vi "Manual.vi"(8 "error in (no error)":errorcluster, 10 "shutdown":refnum<user-event>, 11 "Modules":T2) -> (0 "Error 2":errorcluster)   [LabVIEW 2025]
uses:
  <vilib>/Handler Framework/CmdQueue/Enqueue Single.vi
  <vilib>/Handler Framework/Handler Framework.lvlib
  Libraries/USB IO/USB IO.lvlib
  Libraries/Wheatstone Bridge/Wheatstone Bridge.lvlib
  Libraries/Motor/Motor.lvlib
  Controls/Waveform Chart.ctl
panel:
  in  "Unit Power":bool
  in  "Brake Disable":bool
  in  "Position":dbl min=0.0 max=180.0
  out "Waveform Chart":T1
  out "Angle":dbl format="%5.3f°"
  out "Torque":dbl format="%5.3f lb-in"
  in  "Clear Motor Error":bool
  out "error out":errorcluster
  out "Module Names":string[](array[string])
  out "Error":errorcluster
  # "Manual"
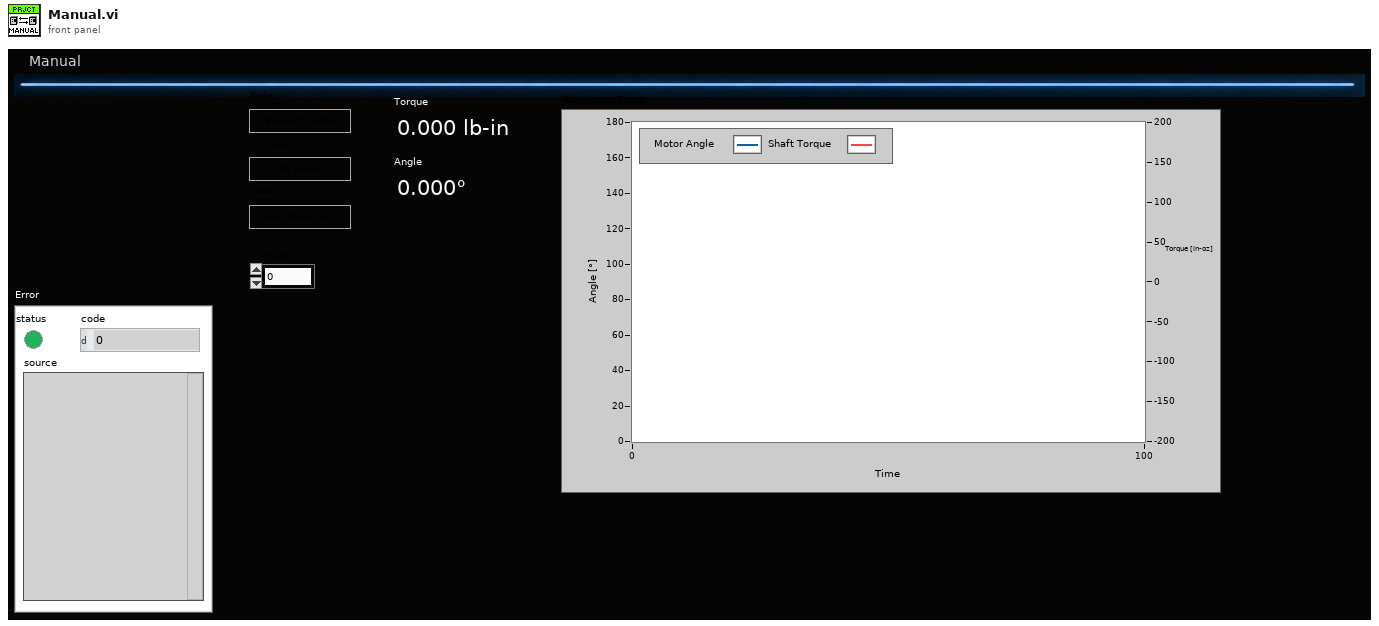
[diagram p1: front panel]
types:
  T1 = typedef "Waveform Chart.ctl" = dbl
  T2 = cluster{"Module IDs":i32[], "Module Names":string[]}
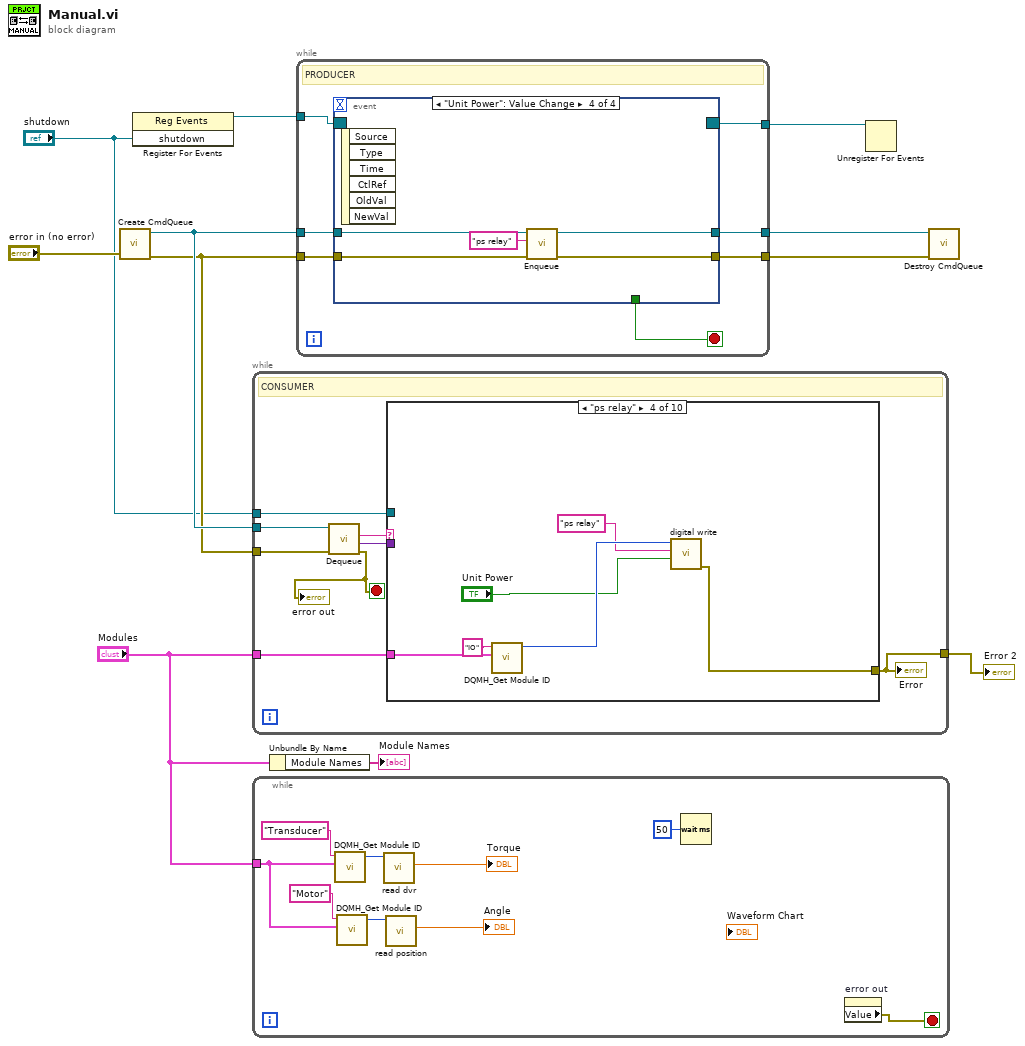
[diagram p0: block diagram]
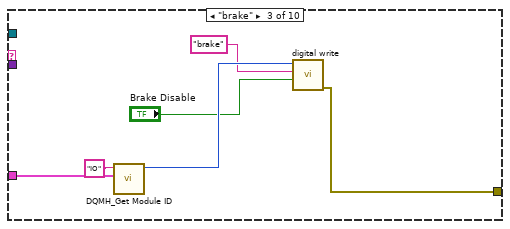
[diagram p4: hidden frame]
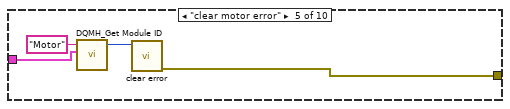
[diagram p5: hidden frame]
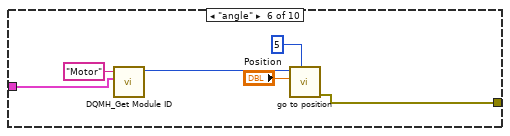
[diagram p6: hidden frame]
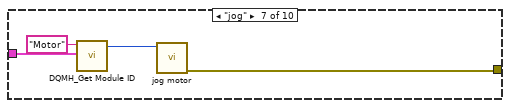
[diagram p7: hidden frame]
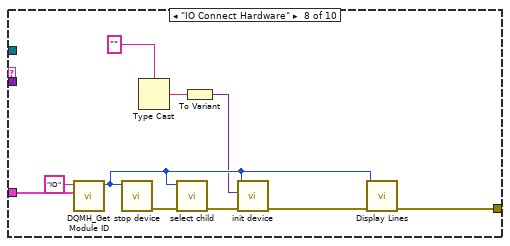
[diagram p8: hidden frame]
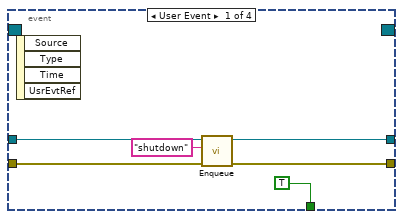
[diagram p11: hidden frame]
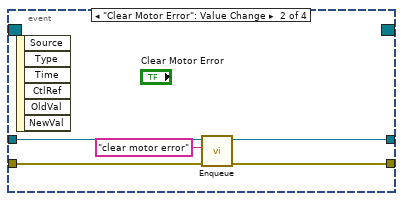
[diagram p12: hidden frame]
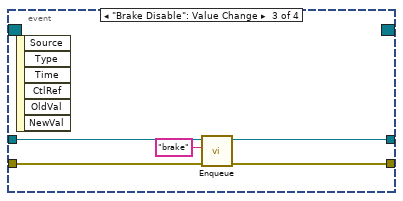
[diagram p13: hidden frame]
diagram:
  n1 = call <vilib>:"Create CmdQueue.vi"("error in (no error)"="error in (no error)") -> ("error out"=w8:errorcluster, "CmdQueue out"=w9:refnum<queue>)  [unwired: 9 in]
  n2 = register-events("shutdown") -> (reference out=w7:refnum<event-registration>)  [unwired: 2 in, 1 out]
  n3 = while {
    tunnel: w9 -> [w19]
    tunnel: w8 -> [w15]
    tunnel: "shutdown" -> [w14]
    tunnel: "Modules" -> [w13]
    tunnel: [w12] -> w2
    stop <- w16 stop-if-true
    # "CONSUMER"
    n4 = call <vilib>:"Dequeue.vi"("error in (no error)"=w15, "CmdQueue in"=w19) -> ("error out"=w16:errorcluster, "value"=w17:variant, "cmd"=w18:string)  [unwired: 5 in, 2 out]
    "error out" <- w16
    n5 = case shown="\"ps relay\"" w18 {
      tunnel: w17 -> [_ _ _ _ _ _ _ _ _ _]
      tunnel: w14 -> [_ _ _ _ _ _ _ _ _ _]
      tunnel: w13 -> [_ _ w24 w30 w34 w40 w45 w55 _ _]
      tunnel: [_ _ w22 w28 w32 w38 w42 w46 _ _] -> w12
      frame "False", Default {
      }
      frame "init" {
      }
      frame "brake" {
        n6 = call "DQMH_Get Module ID.vi"("Modules"=w24, "Module Name"="IO") -> ("Module ID out"=w23:i32)  [unwired: 9 in]
        n7 = call "digital write.vi"("On/Off"="Brake Disable", "Line"="brake", "Module ID"=w23) -> ("error out"=w22:errorcluster)  [unwired: 7 in, 1 out]
      }
      frame "ps relay" {
        n8 = call "DQMH_Get Module ID.vi"("Modules"=w30, "Module Name"="IO") -> ("Module ID out"=w29:i32)  [unwired: 9 in]
        n9 = call "digital write.vi"("On/Off"="Unit Power", "Line"="ps relay", "Module ID"=w29) -> ("error out"=w28:errorcluster)  [unwired: 7 in, 1 out]
      }
      frame "clear motor error" {
        n10 = call "DQMH_Get Module ID.vi"("Modules"=w34, "Module Name"="Motor") -> ("Module ID out"=w33:i32)  [unwired: 9 in]
        n11 = call "clear error.vi"("Module ID"=w33) -> ("error out"=w32:errorcluster)  [unwired: 9 in, 1 out]
      }
      frame "angle" {
        n12 = call "DQMH_Get Module ID.vi"("Modules"=w40, "Module Name"="Motor") -> ("Module ID out"=w39:i32)  [unwired: 9 in]
        n13 = call "go to position.vi"("Pause Time [ms]"=5, "Position"="Position", "Module ID"=w39) -> ("error out"=w38:errorcluster)  [unwired: 6 in, 2 out]
      }
      frame "jog" {
        n14 = call "DQMH_Get Module ID.vi"("Modules"=w45, "Module Name"="Motor") -> ("Module ID out"=w43:i32)  [unwired: 9 in]
        n15 = call "jog motor.vi"("Module ID"=w43) -> ("error out"=w42:errorcluster)  [unwired: 8 in, 2 out]
      }
      frame "IO Connect Hardware" {
        n16 = call "DQMH_Get Module ID.vi"("Modules"=w55, "Module Name"="IO") -> ("Module ID out"=w53:i32)  [unwired: 9 in]
        n17 = call "stop device.vi"("Module ID"=w53) -> ("error out"=w49:errorcluster)  [unwired: 9 in, 1 out]
        n18 = Type Cast(type="") -> (*(type *) &x=w51:string)  [unwired: 1 in]
        n19 = call "select child.vi"("error in"=w49, "Module ID"=w53) -> ("error out"=w47:errorcluster)  [unwired: 8 in, 1 out]
        n20 = To Variant(anything=w51) -> (Variant=w50:variant)
        n21 = call "init device.vi"("error in"=w47, "Variant"=w50, "Module ID"=w53) -> ("error out"=w48:errorcluster)  [unwired: 7 in, 1 out]
        n22 = call "Display Lines.vi"("error in"=w48, "Module ID"=w53) -> ("error out"=w46:errorcluster)  [unwired: 6 in, 3 out]
      }
      frame "Read Voltage" {
      }
      frame "shutdown" {
      }
    }
    "Error" <- w12
  }
  "Error 2" <- w2
  n23 = while {
    tunnel: "Modules" -> [w58]
    stop <- w62 stop-if-true
    n24 = call "DQMH_Get Module ID.vi"("Modules"=w58, "Module Name"="Transducer") -> ("Module ID out"=w63:i32)  [unwired: 9 in]
    n25 = call "DQMH_Get Module ID.vi"("Modules"=w58, "Module Name"="Motor") -> ("Module ID out"=w57:i32)  [unwired: 9 in]
    n26 = call "read dvr.vi"("Module ID"=w63) -> ("Numeric"=→"Torque":dbl)  [unwired: 8 in, 2 out]
    n27 = call "read position.vi"("Module ID"=w57) -> ("Position"=→"Angle":dbl)  [unwired: 8 in, 2 out]
    n28 = Wait (ms)(milliseconds to wait=u32 50) -> ()  [unwired: 1 out]
    n29 = property on="error out" class="Clust (strict)"() -> ("Value"=w62:errorcluster)  [unwired: 2 in, 2 out]
  }
  n30 = Unbundle By Name("Modules") -> ("Module Names"=→"Module Names":string[])
  n31 = while {
    tunnel: w9 -> [w71]
    tunnel: [w70] -> w11
    tunnel: w8 -> [w69]
    tunnel: [w68] -> w10
    tunnel: w7 -> [w66]
    tunnel: [w65] -> w6
    stop <- w67 stop-if-true
    # "PRODUCER"
    n32 = event shown="[3] \"Unit Power\": Value Change" {
      selector: w66 -> [_ _ _ _]
      dyn-events: [_ _ _ _] -> w65
      timeout: _ -> [_ _ _ _]
      tunnel: w71 -> [w77 w82 w87 w92]
      tunnel: [w76 w81 w86 w91] -> w70
      tunnel: w69 -> [w75 w80 w85 w90]
      tunnel: [w74 w79 w84 w89] -> w68
      tunnel: [TRUE ("Discard?") _ _ _] -> w67
      event User Event {
        n33 = event-data() -> ()  [unwired: 1 in, 4 out]
        n34 = call-poly <vilib>:"Enqueue.vi"("error in (no error)"=w75, "Command"="shutdown", "CmdQueue in"=w77) -> ("error out"=w74:errorcluster, "CmdQueue out"=w76:refnum<queue>)  [unwired: 7 in]
      }
      event "Clear Motor Error": Value Change {
        n35 = event-data() -> ()  [unwired: 1 in, 6 out]
        n36 = call-poly <vilib>:"Enqueue.vi"("error in (no error)"=w80, "Command"="clear motor error", "CmdQueue in"=w82) -> ("error out"=w79:errorcluster, "CmdQueue out"=w81:refnum<queue>)  [unwired: 7 in]
      }
      event "Brake Disable": Value Change {
        n37 = event-data() -> ()  [unwired: 1 in, 6 out]
        n38 = call-poly <vilib>:"Enqueue.vi"("error in (no error)"=w85, "Command"="brake", "CmdQueue in"=w87) -> ("error out"=w84:errorcluster, "CmdQueue out"=w86:refnum<queue>)  [unwired: 7 in]
      }
      event "Unit Power": Value Change {
        n39 = event-data() -> ()  [unwired: 1 in, 6 out]
        n40 = call-poly <vilib>:"Enqueue.vi"("error in (no error)"=w90, "Command"="ps relay", "CmdQueue in"=w92) -> ("error out"=w89:errorcluster, "CmdQueue out"=w91:refnum<queue>)  [unwired: 7 in]
      }
    }
  }
  n41 = Unregister For Events(event registration refnum=w6) -> ()  [unwired: 1 in, 1 out]
  n42 = call <vilib>:"Destroy CmdQueue.vi"("error in (no error)"=w10, "CmdQueue in"=w11) -> ()  [unwired: 9 in, 1 out]
